vi "All Watchdog Manager.vi"(8 "error in (no error)":errorcluster, 10 "Infinite Message Selector":T1, 11 "Guardian in":refnum<class "Guardian.lvclass">) -> (0 "error out":errorcluster, 2 "Status":bool, 3 "Guardian out":refnum<class "Guardian.lvclass">)   [LabVIEW 2026, in "TALOS.lvlib" / "Guardian.lvlib" / "Guardian.lvclass"]
uses:
  Guardian.lvclass
  Ancestor/Ancestor/Infinite Message Selector.ctl
  a2f3f938-3bec-452b-b06c-bc4e00b2b752.vi
  Ancestor/Ancestor/Ancestor.lvclass
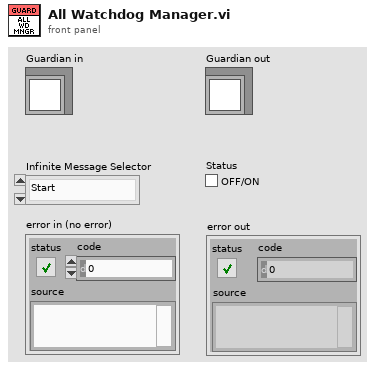
[diagram p1: front panel]
types:
  T1 = typedef "TALOS.lvlib/Ancestor.lvlib/Ancestor.lvclass/Infinite Message Selector.ctl" = enum16{"Start", "Stop", "Check", "Flush (Stop all)", "Init"}
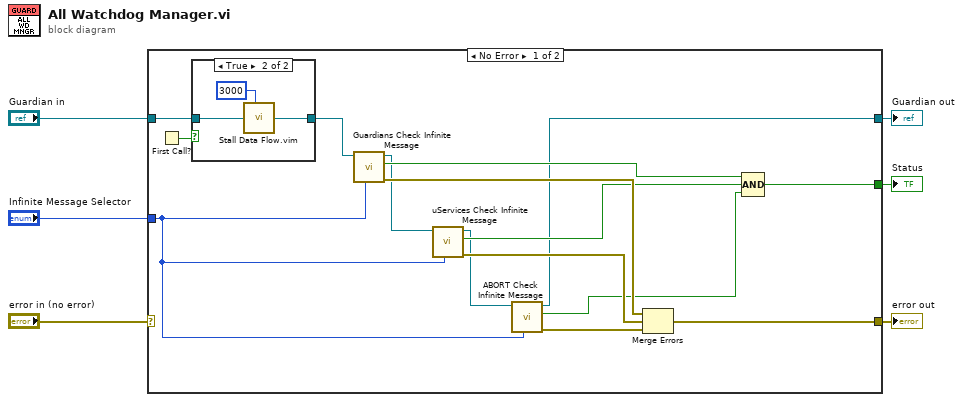
[diagram p0: block diagram]
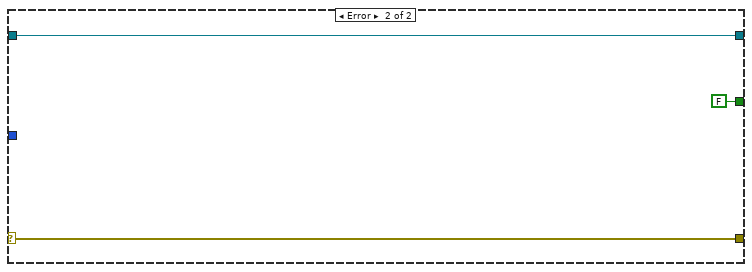
[diagram p3: hidden frame]
diagram:
  n1 = case shown="No Error" "error in (no error)" {
    selector: "error in (no error)" -> [_ w28]
    tunnel: [w9 w27] -> w6
    tunnel: "Guardian in" -> [w20 w27]
    tunnel: [w19 w28] -> w4
    tunnel: "Infinite Message Selector" -> [w16 _]
    tunnel: [w7 FALSE] -> w1
    frame No Error {
      n2 = First Call?() -> (First Call?: T/F=w14:bool)
      n3 = case shown="True" w14 {
        tunnel: w20 -> [w22 w25]
        tunnel: [w22 w24] -> w15
        frame False {
        }
        frame True {
          n4 = call "Stall Data Flow.vim"("value in"=w25, "milliseconds to wait"=u32 3000) -> ("value out"=w24:refnum<class "Guardian.lvclass">)  [unwired: 1 out]
        }
      }
      n5 = call "Guardians Check Infinite Message.vi"("Infinite Message Selector"=w16, "Guardian in"=w15) -> ("error out"=w18:errorcluster, "Exists?"=w13:bool, "Guardian out"=w11:refnum<class "Guardian.lvclass">)  [unwired: 7 in]
      n6 = call "uServices Check Infinite Message.vi"("Infinite Message Selector"=w16, "Guardian in"=w11) -> ("error out"=w17:errorcluster, "Exists?"=w12:bool, "Guardian out"=w10:refnum<class "Guardian.lvclass">)  [unwired: 7 in]
      n7 = call "ABORT Check Infinite Message.vi"("Infinite Message Selector"=w16, "Guardian in"=w10) -> ("error out"=w21:errorcluster, "Exists?"=w8:bool, "Guardian out"=w9:refnum<class "Guardian.lvclass">)  [unwired: 7 in]
      n8 = Merge Errors(w18, w17, w21) -> (w19:errorcluster)
      n9 = Compound Arithmetic op=AND(w13, w12, w8) -> (w7:bool)
    }
    frame Error {
    }
  }
  "error out" <- w4
  "Guardian out" <- w6
  "Status" <- w1
